vi "LVClass_ModalCoef Save To File.vi"(0 "ModalCoef in":refnum<class "ModalCoef.lvclass">, 5 "coefs_file_path":path, 7 "comments":string, 11 "error in (no error)":errorcluster) -> (4 "ModalCoef out":refnum<class "ModalCoef.lvclass">, 15 "error out":errorcluster)   [LabVIEW 2020, in "ModalCoef.lvclass"]
doc: "ModalCoef constructor.\n\n--------------------------------------------------------------------------------\n\n<B>ModalCoefIn </B> : Constant Pointer to ModalCoef object.\n<B>ModalCoefOut </B> : Constant Pointer to ModalCoef object.\n<B>TypePhase </B> : TypePhase Phase mode reconstruction.\n<B>ErrorIn </B> : Error\n<B>ErrorOut </B> : Error\n\n--------------------------------------------------------------------------------"
uses:
  ModalCoef.lvclass
  ModalCoef.lvclass/ModalCoef.ctl
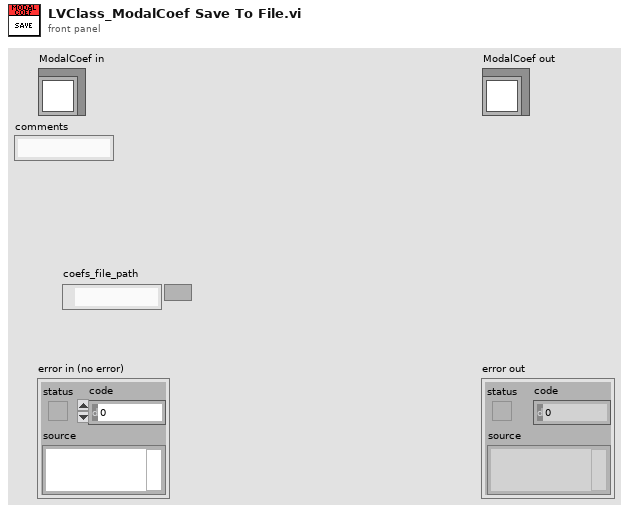
[diagram p1: front panel]
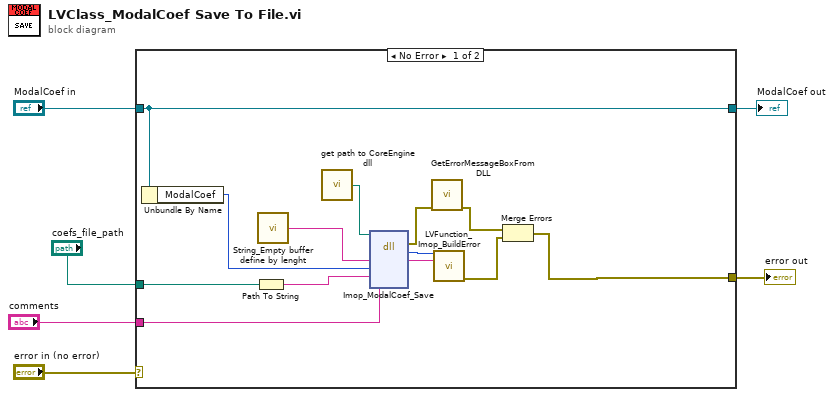
[diagram p0: block diagram]
diagram:
  n1 = case shown="No Error" "error in (no error)" {
    selector: "error in (no error)" -> [_ w21]
    tunnel: [w12 w21] -> w5
    tunnel: [w8 w20] -> w3
    tunnel: "ModalCoef in" -> [w8 w20]
    tunnel: "coefs_file_path" -> [w11 _]
    tunnel: "comments" -> [w7 _]
    frame No Error {
      n2 = Unbundle By Name(w8) -> ("ModalCoef"=w9:i32)
      n3 = Path To String(path=w11) -> (string=w10:string)
      n4 = call "String_Empty buffer define by lenght.vi"() -> ("Empty buffer"=w19:string)  [unwired: 1 in]
      n5 = call "get path to CoreEngine dll.vi"() -> ("path to c_interface_vc100.dll"=w16:path)  [unwired: 12 in, 3 out]
      n6 = dll-call lib="D:/soft/HASO_v3/SVN_trunk/ImOpCoreEngine4_LV2011/DLLs/c_interface_vc100.dll" fn="Imop_ModalCoef_Save"(path in=w16, "message"=w19, "ModalCoef"=w9, "coefs_file_path"=w10, "comments"=w7) -> (error out=w15:errorcluster, "return type"=w17:i32, "message"=w18:string)  [unwired: 5 in, 1 out]
      n7 = call "GetErrorMessageBoxFromDLL.vi"("error IN"=w15) -> ("error OUT"=w14:errorcluster)  [unwired: 10 in]
      n8 = call "LVFunction_Imop_BuildError.vi"("code"=w17, "String to Prepend to source (\"\")"=w18) -> ("error out"=w13:errorcluster)  [unwired: 13 in]
      n9 = Merge Errors(w14, w13) -> (w12:errorcluster)
    }
    frame Error {
    }
  }
  "error out" <- w5
  "ModalCoef out" <- w3
